vi "find all instances with alias.vi"(10 "Alias":string, 11 "flat hierarchy":T2) -> (3 "instance data":T1[](array[typedef]))   [LabVIEW 2025, in "CEF.lvlib"]
doc: "Finds all instances in a flattened instance data set which have a given alias.Copyright 2017 National Instruments Corporation\n\nLicensed under the Apache License, Version 2.0 (the \"License\"); you may not use this file except in compliance with the License. You may obtain a copy of the License at http://www.apache.org/licenses/LICENSE-2.0\nUnless required by applicable law or agreed to in writing, software distributed under the License is distributed on an \"AS IS\" BASIS, WITHOUT WARRANTIES OR CONDITIONS OF ANY KIND, either express or implied. See the License for the specific language governing permissions and limitations under the License."
uses:
  CEF.lvlib
  flat hierarchy.ctl
  hierarchy repo/full hierarchy.ctl
  hierarchy element.ctl
  instance data.ctl
  hierarchy repo/CEF_HierarchyRepo.lvclass
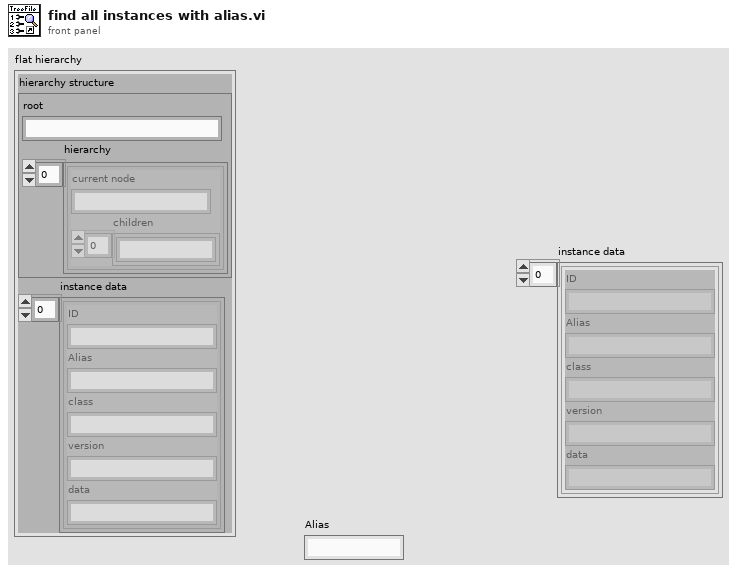
[diagram p1: front panel]
types:
  T1 = typedef "CEF.lvlib/instance data.ctl" = cluster{"ID":string, "Alias":string, "class":string, "version":string, "data":string}
  T2 = typedef "CEF.lvlib/flat hierarchy.ctl" = cluster{"hierarchy structure":T3, "instance data":T1[]}
  T3 = typedef "CEF.lvlib/CEF_HierarchyRepo.lvclass/full hierarchy.ctl" = cluster{"root":string, "hierarchy":T4[]}
  T4 = typedef "CEF.lvlib/hierarchy element.ctl" = cluster{"current node":string, "children":string[]}
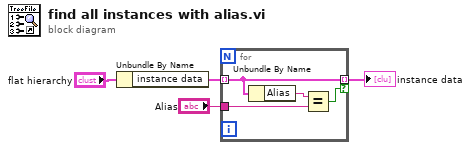
[diagram p0: block diagram]
diagram:
  n1 = Unbundle By Name("flat hierarchy") -> ("instance data"=w3:T1[])
  n2 = for {
    tunnel: w3 -> [w6] mode=indexing
    tunnel: "Alias" -> [w8]
    tunnel: [w6] -> w1 mode=indexing if=w5
    n3 = Unbundle By Name(w6) -> ("Alias"=w7:string)
    n4 = Equal?(x=w7, y=w8) -> (x = y?=w5:bool)
  }
  "instance data" <- w1
